vi "Test Seek Position WAV.vi"(8 "error in (no error)":errorcluster) -> (0 "error out":errorcluster, 3 "Pass?":bool)   [LabVIEW 2020]
uses:
  G-Audio/Private/Result To Error.vi
  <vilib>/Utility/error.llb/Error Cluster From Error Code.vi
  G-Audio/G-Audio.lvlib
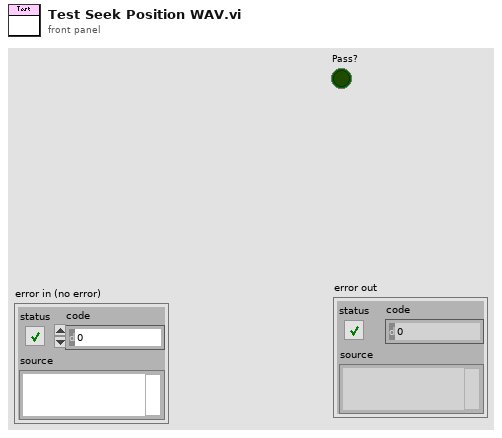
[diagram p1: front panel]
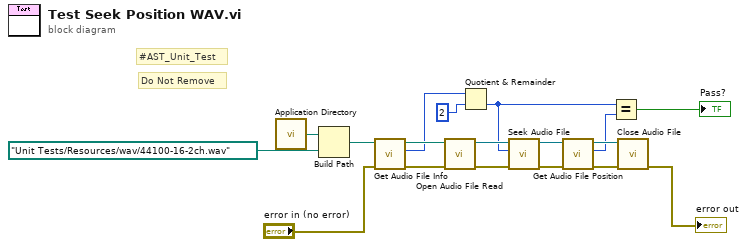
[diagram p0: block diagram]
diagram:
  # "Do Not Remove"
  # "#AST_Unit_Test"
  n1 = call <vilib>:"Application Directory.vi"() -> ("Application Directory"=w13:path)
  n2 = Build Path(base path=w13, name or relative path=path "Unit Tests/Resources/wav/44100-16-2ch.wav" ("Path")) -> (appended path=w11:path)
  n3 = call "Get Audio File Info.vi"("error in (no error)"="error in (no error)", "Path In"=w11) -> ("error out"=w17:errorcluster, "PCM Frame Length"=w9:u64, "Path Out"=w10:path)  [unwired: 6 in, 1 out]
  n4 = call "Open Audio File Read.vi"("error in (no error)"=w17, "Path"=w10) -> ("error out"=w16:errorcluster, "Audio File Refnum"=w18:refnum<file>)  [unwired: 8 in]
  n5 = Quotient & Remainder(x=w9, y=u64 2) -> (floor(x/y)=w2:u64)  [unwired: 1 out]
  n6 = call "Seek Audio File.vi"("error in (no error)"=w16, "Frame Position"=w2, "Audio File Refnum In"=w18) -> ("error out"=w15:errorcluster, "Audio File Refnum Out"=w5:refnum<file>)  [unwired: 7 in]
  n7 = call "Get Audio File Position.vi"("error in (no error)"=w15, "Audio File Refnum In"=w5) -> ("error out"=w6:errorcluster, "Frame Position"=w3:u64, "Audio File Refnum Out"=w4:refnum<file>)  [unwired: 7 in]
  n8 = Equal?(x=w2, y=w3) -> (x = y?=→"Pass?":bool)
  n9 = call "Close Audio File.vi"("error in (no error)"=w6, "Audio File Refnum In"=w4) -> ("error out"=→"error out":errorcluster)  [unwired: 9 in]
